vi "MsgParser.vi"(2 "LAST MSGS":refnum<vi>, 3 "MSG LOG":refnum<vi>, 4 "MSG Counter":i32, 5 "current msg num":i32) -> (0 "Result Counter":i32)   [LabVIEW 2010]
panel:
  in  "VOC Last Interation MSG":i32(listbox)
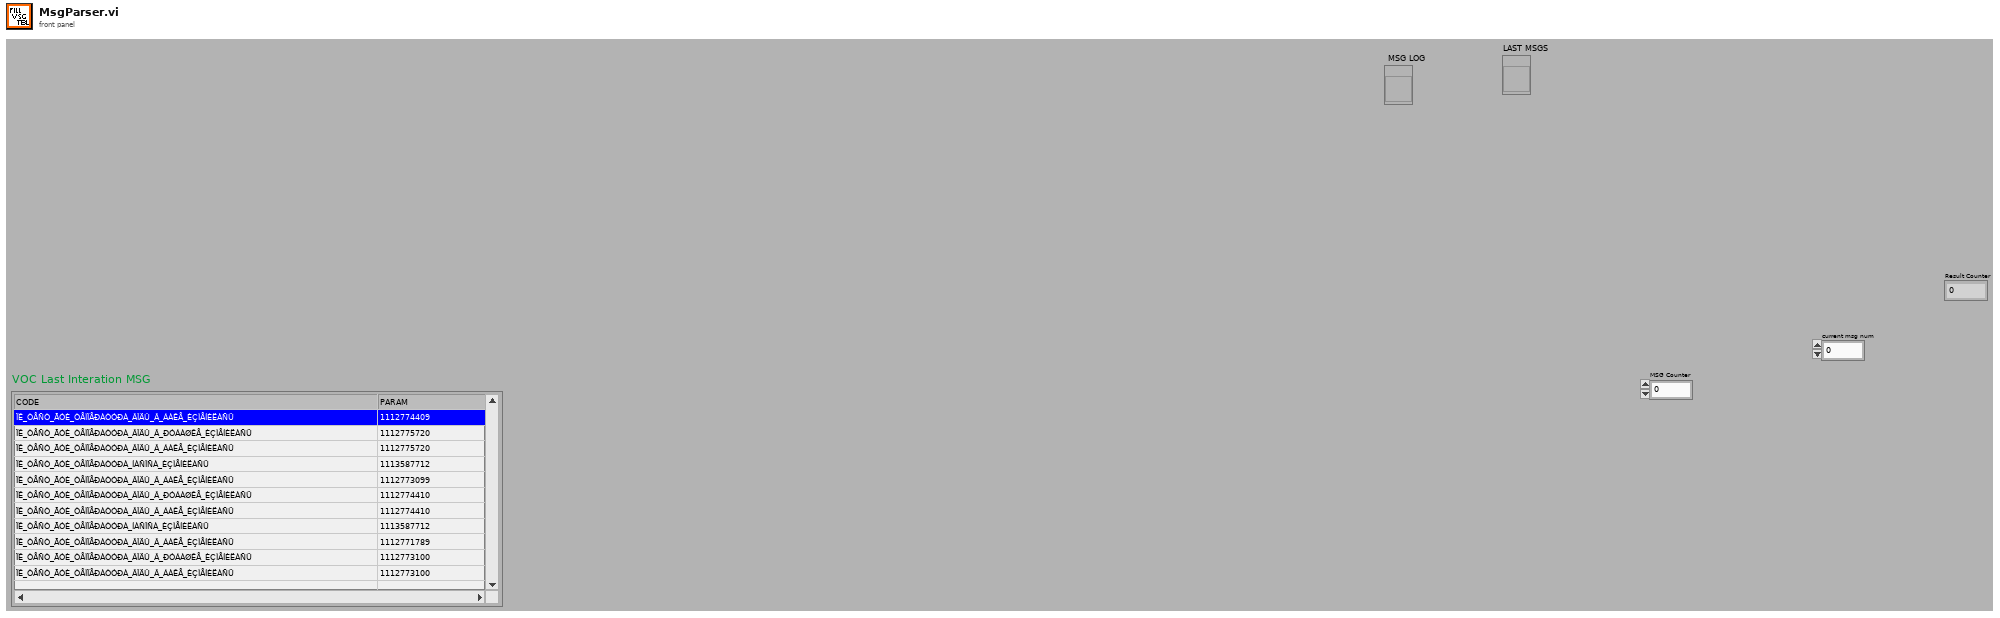
[diagram p1: front panel]
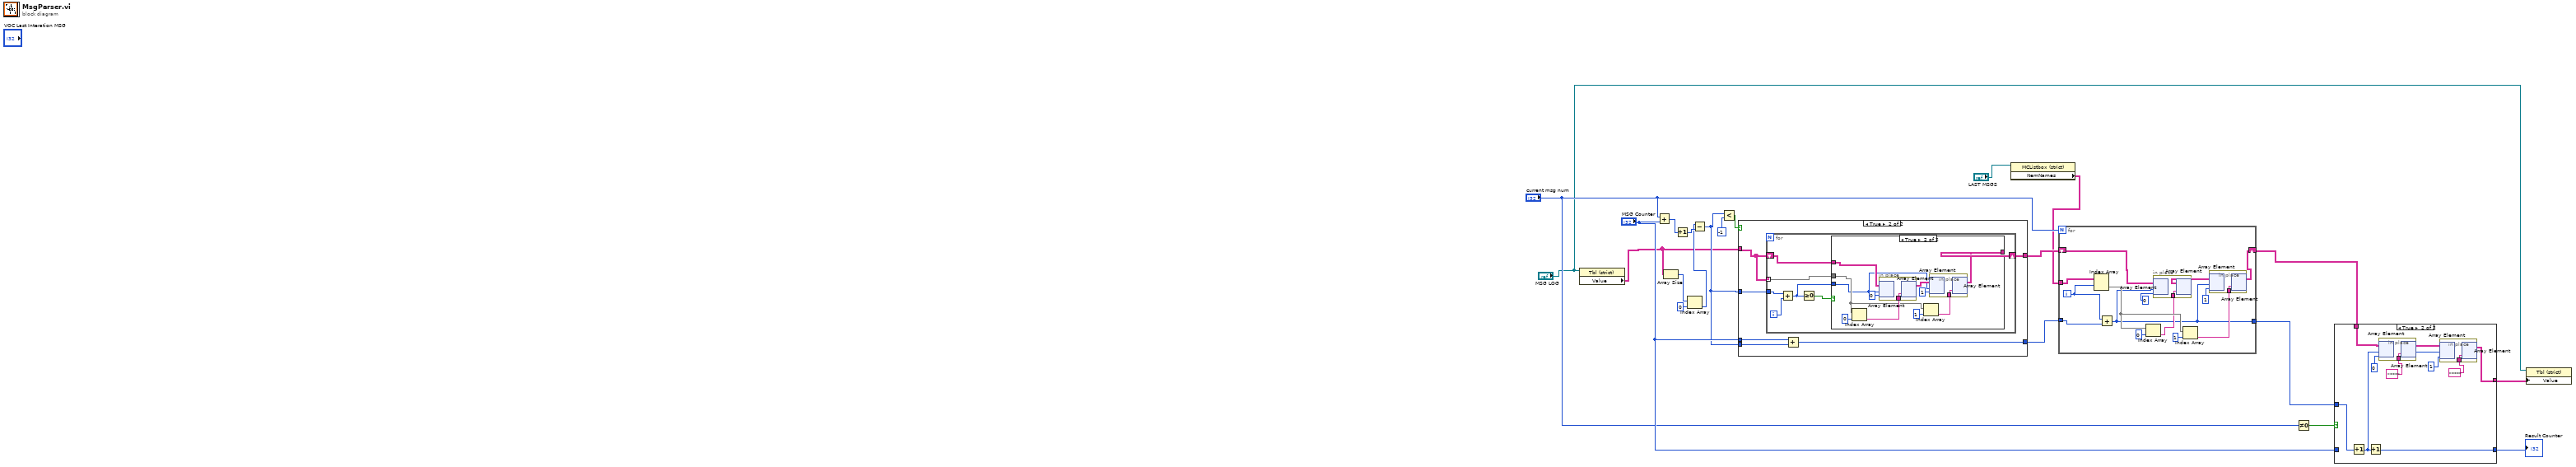
[diagram p0: block diagram]
diagram:
  n1 = property class="Tbl (strict)"(reference="MSG LOG") -> ("Value"=w6:string[][])  [unwired: 1 in, 2 out]
  n2 = Add(x="current msg num", y="MSG Counter") -> (x+y=w18:i32)
  n3 = Array Size(array=w6) -> (size(s)=w9:i32[])
  n4 = Increment(x=w18) -> (x+1=w17:i32)
  n5 = Index Array(array=w9, index=0) -> (element=w7:i32)
  n6 = Subtract(x=w7, y=w17) -> (x-y=w16:i32)
  n7 = Less?(x=w16, y=-1) -> (x < y?=w14:bool)
  n8 = case shown="True" w14 {
    tunnel: w6 -> [w23 w24]
    tunnel: w16 -> [_ w29]
    tunnel: w16 -> [_ w26]
    tunnel: [w23 w28] -> w13
    tunnel: "MSG Counter" -> [w22 w27]
    tunnel: [w22 w25] -> w11
    frame False {
    }
    frame True {
      n9 = for {
        shift-right: [w34] -> w28
        shift-left: w24 -> [w36]
        tunnel: w24 -> [w35] mode=indexing
        tunnel: w29 -> [w33]
        i -> [w31]
        n10 = Add(x=w33, y=w31) -> (x+y=w30:i32)
        n11 = Greater Or Equal To 0?(x=w30) -> (x >= 0?=w32:bool)
        n12 = case shown="True" w32 {
          tunnel: w36 -> [w37 w39]
          tunnel: w35 -> [_ w41]
          tunnel: [w37 w44] -> w34
          tunnel: w30 -> [_ w38]
          frame False {
          }
          frame True {
            n13 = Index Array(array=w41, index=0) -> (element=w46:string)
            n14 = in-place {
              in-place-border: w46 -> [w50]
              n15 = in-place-array #1(w39, w38, 0) -> ()  [unwired: 1 out]
              n16 = in-place-array #1(w50) -> (w45:string[][])  [unwired: 2 out]
            }
            n17 = Index Array(array=w41, index=1) -> (element=w40:string)
            n18 = in-place {
              in-place-border: w40 -> [w49]
              n19 = in-place-array #2(w45, w38, 1) -> ()  [unwired: 1 out]
              n20 = in-place-array #2(w49) -> (w44:string[][])  [unwired: 2 out]
            }
          }
        }
      }
      n21 = Add(x=w27, y=w26) -> (x+y=w25:i32)
    }
  }
  n22 = property class="MCListbox (strict)"(reference="LAST MSGS") -> ("ItemNames"=w4:string[][])  [unwired: 1 in, 2 out]
  n23 = for {
    N: "current msg num" -> [_]
    shift-right: [w51] -> w2
    shift-left: w13 -> [w58]
    tunnel: w4 -> [w64]
    tunnel: w11 -> [w62]
    tunnel: [w52] -> w10
    i -> [w63]
    n24 = Index Array(array=w64, index (row)=w63) -> (element=w55:string[])  [unwired: 1 in]
    n25 = Add(x=w63, y=w62) -> (x+y=w52:i32)
    n26 = Index Array(array=w55, index=0) -> (element=w54:string)
    n27 = in-place {
      in-place-border: w54 -> [w66]
      n28 = in-place-array #3(w58, w52, 0) -> ()  [unwired: 1 out]
      n29 = in-place-array #3(w66) -> (w60:string[][])  [unwired: 2 out]
    }
    n30 = Index Array(array=w55, index=1) -> (element=w53:string)
    n31 = in-place {
      in-place-border: w53 -> [w65]
      n32 = in-place-array #4(w60, w52, 1) -> ()  [unwired: 1 out]
      n33 = in-place-array #4(w65) -> (w51:string[][])  [unwired: 2 out]
    }
  }
  n34 = Not Equal To 0?(x="current msg num") -> (x != 0?=w20:bool)
  n35 = case shown="True" w20 {
    tunnel: w10 -> [_ w79]
    tunnel: w2 -> [w68 w77]
    tunnel: [w68 w69] -> w1
    tunnel: [w67 w78] -> w21
    tunnel: "MSG Counter" -> [w67 _]
    frame False {
    }
    frame True {
      n36 = Increment(x=w79) -> (x+1=w76:i32)
      n37 = Increment(x=w76) -> (x+1=w78:i32)
      n38 = in-place {
        in-place-border: "***" ("new element/subarray") -> [w81]
        n39 = in-place-array #5(w77, w76, 0 ("disabled index (col)")) -> ()  [unwired: 1 out]
        n40 = in-place-array #5(w81) -> (w73:string[][], w72:i32)  [unwired: 1 out]
      }
      n41 = in-place {
        in-place-border: "***" ("new element/subarray") -> [w80]
        n42 = in-place-array #6(w73, w72, 1 ("disabled index (col)")) -> ()  [unwired: 1 out]
        n43 = in-place-array #6(w80) -> (w69:string[][])  [unwired: 2 out]
      }
    }
  }
  "Result Counter" <- w21
  n44 = property class="Tbl (strict)"(reference="MSG LOG", "Value"=w1) -> ()  [unwired: 1 in, 2 out]
